vi "Example_LEDToggle.vi"() -> ()   [LabVIEW 2021, in "BrainStem2_LabVIEW_Library.lvlib"]
uses:
  BrainStem2_LabVIEW_Library.lvlib
panel:
  out "LED":bool
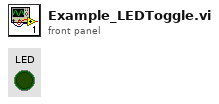
[diagram p1: front panel]
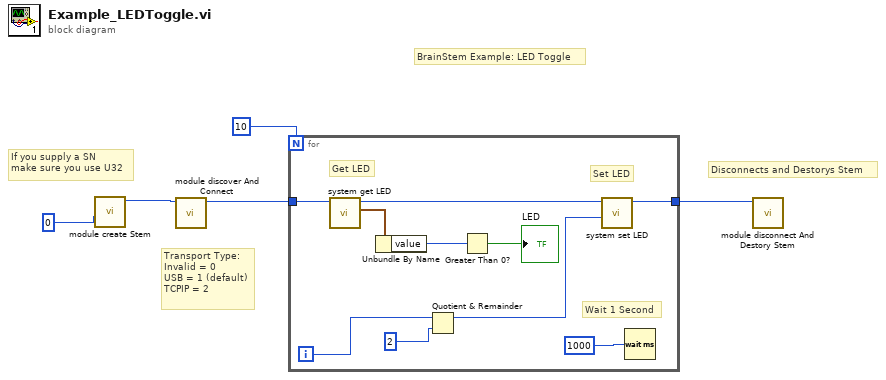
[diagram p0: block diagram]
diagram:
  # "BrainStem Example: LED Toggle"
  # "If you supply a SN\nmake sure you use U32"
  # "Transport Type:\nInvalid = 0\nUSB = 1 (default)\nTCPIP = 2"
  # "Disconnects and Destorys Stem"
  n1 = call "module create Stem.vi"("sn"=u32 0) -> ("id out"=w4:u32)  [unwired: 8 in, 2 out]
  n2 = call "module discover And Connect.vi"("id"=w4) -> ("id out"=w3:u32)  [unwired: 8 in, 2 out]
  n3 = for {
    N: 10 -> [_]
    tunnel: w3 -> [w15]
    tunnel: [w13] -> w2
    i -> [w8]
    # "Wait 1 Second"
    # "Set LED"
    # "Get LED"
    n4 = call "system get LED.vi"("id"=w15) -> ("result out"=w12:cluster{"value":i32, "error":i32}, "id out"=w14:u32)  [unwired: 8 in, 1 out]
    n5 = Unbundle By Name(w12) -> ("value"=w10:i32)
    n6 = Quotient & Remainder(x=w8, y=2) -> (x-y*floor(x/y)=w7:i32)  [unwired: 1 out]
    n7 = Greater Than 0?(x=w10) -> (x > 0?=→"LED":bool)
    n8 = call "system set LED.vi"("bOn"=w7, "id"=w14) -> ("id out"=w13:u32)  [unwired: 7 in, 2 out]
    n9 = Wait (ms)(milliseconds to wait=1000) -> ()  [unwired: 1 out]
  }
  n10 = call "module disconnect And Destory Stem.vi"("id"=w2) -> ()  [unwired: 8 in, 3 out]
